vi "Match_by_best_fit.vi"(1 "ReferenceSessionDataSet":T1[](array[typedef]), 5 "CurrentSessionDataSet":T1[](array[typedef])) -> (0 "Results Out":i32[][](array[numeric]), 2 "Array":i32[](array[numeric]), 3 "IndexRefrenceSession 3":i32[][](array[numeric]), 4 "Array 2":dbl[](array[numeric]), 6 "Boolean":bool, 7 "IndexRefrenceSession":i32[](array[numeric]), 8 "Numeric 2":dbl, 9 "IndexRefrenceSession 2":i32[](array[numeric]), 10 "Numeric":i32)   [LabVIEW 2011]
doc: "Find the best match of the reference session and current session fiducials through geometric test of what rotation or reflection and rotation after scaling produces the least error of the sum of the nearest fiducials. May be a good diagnostic method. Not fully validated."
uses:
  cm2nm_coordinate_information_v2.ctl
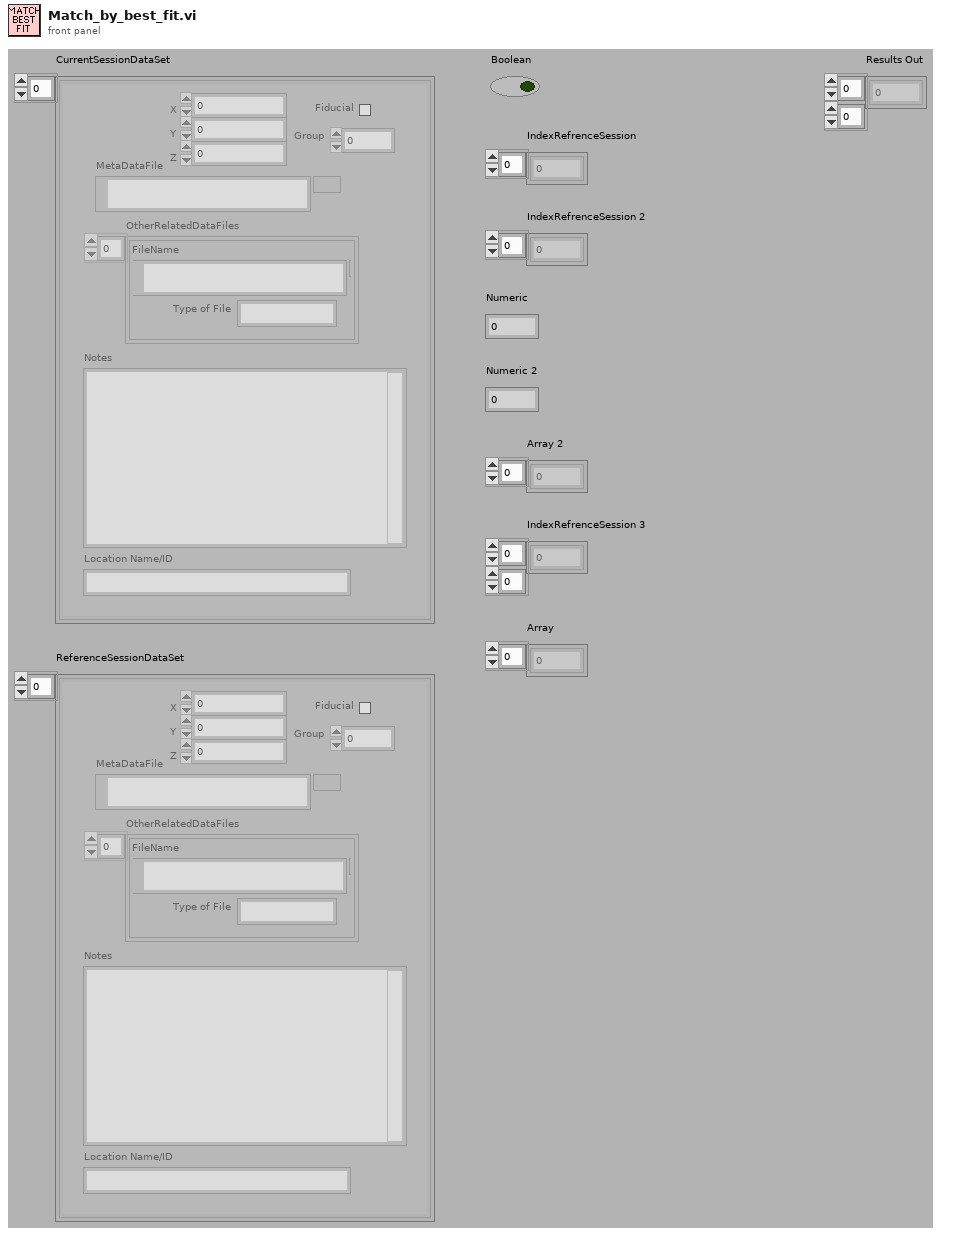
[diagram p1: front panel]
types:
  T1 = typedef "cm2nm_coordinate_information_v2.ctl" = cluster{"MetaDataFile":path, "X":dbl, "Y":dbl, "Z":dbl, "Group":i32, "Rotation":dbl[unit], "Fiducial":bool, "Magnification":dbl, "Working_Distance":dbl, "Notes":string, "Location Name/ID":string, "OtherRelatedDataFiles":cluster{"Type of File":string, "FileName":path}[], "Available":bool}
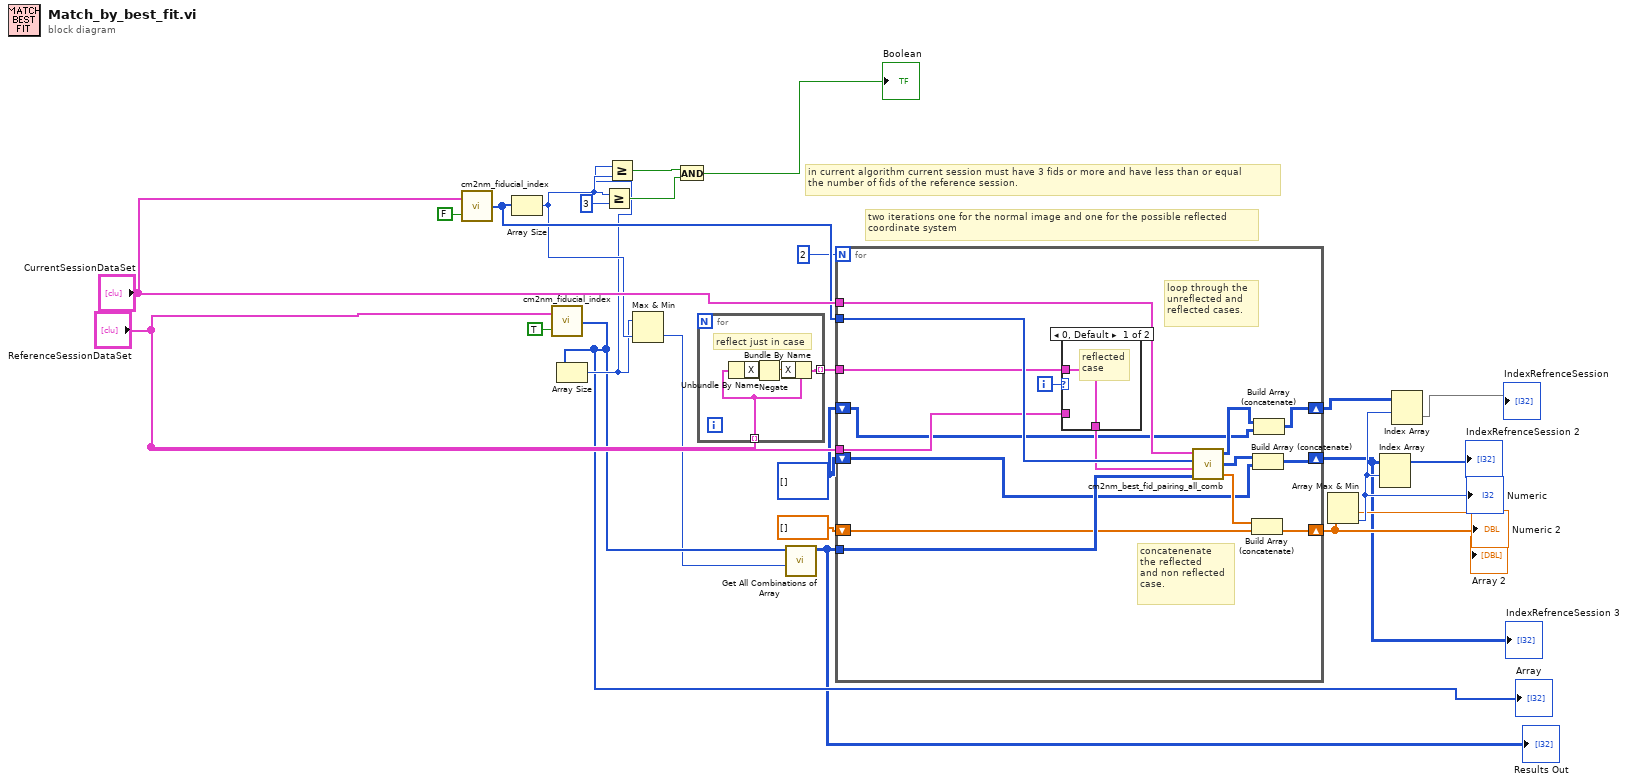
[diagram p0: block diagram]
diagram:
  w22 = i32[][] [] ("IndexRefrenceSession")
  # "in current algorithm current session must have 3 fids or more and have less than or equal \nthe number of fids of the reference session."
  # "two iterations one for the normal image and one for the possible reflected\ncoordinate system"
  n1 = call "cm2nm_fiducial_index.vi"("Accept_unverified"=FALSE, "CollectionOfPoints"="CurrentSessionDataSet") -> ("Array"=w21:i32[])
  n2 = Array Size(array=w21) -> (size(s)=w17:i32)
  n3 = call "cm2nm_fiducial_index.vi"("Accept_unverified"=TRUE, "CollectionOfPoints"="ReferenceSessionDataSet") -> ("Array"=w12:i32[])
  "Array" <- w12
  n4 = Array Size(array=w12) -> (size(s)=w16:i32)
  n5 = Greater Or Equal?(x=w17, y=3) -> (x >= y?=w18:bool)
  n6 = Greater Or Equal?(x=w16, y=w17) -> (x >= y?=w19:bool)
  n7 = Max & Min(x=w16, y=w17) -> (min(x,y)=w8:i32)  [unwired: 1 out]
  n8 = And(x=w19, y=w18) -> (x .and. y?=→"Boolean":bool)
  n9 = for {
    tunnel: "ReferenceSessionDataSet" -> [w28] mode=indexing
    tunnel: [w26] -> w5 mode=indexing
    # "reflect just in case"
    n10 = Unbundle By Name(w28) -> ("X"=w29:dbl)
    n11 = Negate(x=w29) -> (-x=w27:dbl)
    n12 = Bundle By Name(cluster=w28, "X"=w27) -> (w26:T1)
  }
  n13 = call "Get All Combinations of Array.vi"("Combination Length"=w8, "Array"=w12) -> ("Results Out"=w2:i32[][])  [unwired: 7 in, 2 out]
  "Results Out" <- w2
  n14 = for {
    N: 2 -> [_]
    tunnel: "ReferenceSessionDataSet" -> [w40]
    tunnel: "CurrentSessionDataSet" -> [w45]
    tunnel: w21 -> [w44]
    tunnel: w2 -> [w43]
    tunnel: w5 -> [w41]
    shift-right: [w37] -> w3
    shift-left: dbl[] [] -> [w36]
    shift-right: [w33] -> w1
    shift-left: w22 -> [w35]
    shift-right: [w31] -> w13
    shift-left: w22 -> [w30]
    i -> [w42]
    # "concatenenate\nthe reflected\nand non reflected\ncase."
    # "loop through the\nunreflected and\nreflected cases."
    n15 = case shown="0, Default" w42 {
      tunnel: w41 -> [w46 _]
      tunnel: w40 -> [_ w47]
      tunnel: [w46 w47] -> w39
      frame 0, Default {
        # "reflected\ncase"
      }
      frame 1 {
      }
    }
    n16 = call "cm2nm_best_fid_pairing_all_comb.vi"("ReferenceCombinatations"=w43, "ReferenceSessionDataSet"=w39, "CurrentSessionindeces"=w44, "CurrentSessionDataSet"=w45) -> ("Array of the total error"=w38:dbl[], "IndexRefrenceSession"=w34:i32[][], "IndexCurrentSession"=w32:i32[][])
    n17 = Build Array (concatenate)(w38, w36) -> (w37:dbl[])
    n18 = Build Array (concatenate)(w34, w35) -> (w33:i32[][])
    n19 = Build Array (concatenate)(w32, w30) -> (w31:i32[][])
  }
  "Array 2" <- w3
  "IndexRefrenceSession 3" <- w1
  n20 = Array Max & Min(array=w3) -> (min value=→"Numeric 2":dbl, min index (indices)=w14:i32)  [unwired: 2 out]
  "Numeric" <- w14
  n21 = Index Array(array=w1, index (row)=w14) -> (element=→"IndexRefrenceSession 2":i32[])  [unwired: 1 in]
  n22 = Index Array(array=w13, index (row)=w14) -> (element=→"IndexRefrenceSession":i32[])  [unwired: 1 in]
